vi "Get Reference Value.vi"(8 "error in (no error)":errorcluster, 11 "VISA resource name":refnum<visa-resource-name>) -> (0 "error out":errorcluster, 2 "Reference Value":dbl format="%^.3e", 3 "VISA resource name out":refnum<visa-resource-name>)   [LabVIEW 2014, in "Fluke 5XXX Series Multicalibrators.lvlib"]
doc: "This VI returns the present value of the reference when editing the output (error mode). If not editing the output using the FL5XMCAL Change Output Value.vi, the return is 0 (0E+00). The reference value is set with the FL5XMCAL Set Output Values.vi, FL5XMCAL New Reference Value.vi or FL5XMCAL Change Reference Value.vi.\n\nNote:\n\nTo determine which quantity is being edited, use FL5XMCAL Get Edit Field.vi and FL5XMCAL Get Output Values.vi."
uses:
  Fluke 5XXX Series Multicalibrators.lvlib
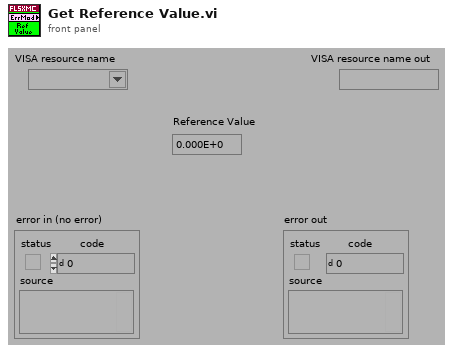
[diagram p1: front panel]
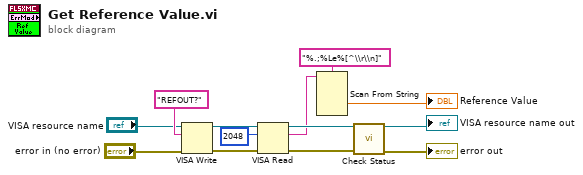
[diagram p0: block diagram]
diagram:
  n1 = VISA Write(VISA resource name="VISA resource name", write buffer="REFOUT?", error in (no error)="error in (no error)") -> (VISA resource name out=w11:refnum<visa-resource-name>, error out=w10:errorcluster)  [unwired: 1 out]
  n2 = VISA Read(VISA resource name=w11, byte count=u32 2048 ("byte count (0)"), error in (no error)=w10) -> (VISA resource name out=w8:refnum<visa-resource-name>, read buffer=w7:string, error out=w9:errorcluster)  [unwired: 1 out]
  n3 = Scan From String(format string="%.;%Le%[^\\r\\n]", input string=w7) -> (output 1=→"Reference Value":dbl)  [unwired: 5 in, 3 out]
  n4 = call "Check Status.vi"("VISA resource name"=w8, "error in (no error)"=w9) -> ("VISA resource name out"=→"VISA resource name out":refnum<visa-resource-name>, "error out"=→"error out":errorcluster)  [unwired: 12 in]
